vi "App_Remove User.vi"(8 "error in":errorcluster) -> (0 "error out":errorcluster)   [LabVIEW 2015, in "Application 1.lvlib"]
uses:
  Application 1.lvlib
  Data Def/App_Main Loop Queue Data.ctl
  Data Def/App_Subpanel Name.ctl
  Data Def/App_User Event Data.ctl
  Data Def/App_Config Method.ctl
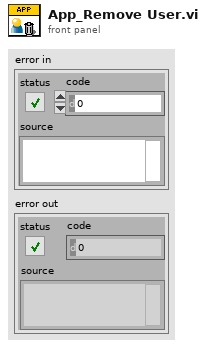
[diagram p1: front panel]
types:
  T1 = typedef "Application 1.lvlib/App_User Event Data.ctl" = cluster{"Command":string, "Data":variant}
  T2 = typedef "Application 1.lvlib/App_Subpanel Name.ctl" = enum16{"Main", "Menu", "User Registering", "User Setting", "Monitor", "Traning Mode", "Query Data", "Connect Setting"}
  T3 = typedef "Application 1.lvlib/App_Config Method.ctl" = enum16{"Get", "Put", "Load", "Save"}
  T4 = typedef "Application 1.lvlib/App_Main Loop Queue Data.ctl" = cluster{"Command":string, "Data":variant}
  T5 = typedef "Application 1.lvlib/App_Main Data.ctl" = cluster{"VI Refnum":refnum<vi>, "Subpanel":refnum<vi>, "Connection ID":refnum<k5>, "Meta data":T6[], "Main Queue":T8, "User Data":T9}
  T6 = typedef "stm_MetaElement.ctl" = cluster{"Name":T7}
  T7 = typedef "stm_MetaDataElement.ctl" = string
  T8 = typedef "Application 1.lvlib/App_Main Queue.ctl" = cluster{"Main Loop Queue":refnum<queue>}
  T9 = typedef "User Data.ctl" = cluster{"Name":string, "Email":string, "Phone Number":string, "User Picture":u32[][], "Last Login Time":timestamp}
  T10 = typedef "Application 1.lvlib/App_Configuration.ctl" = cluster{"Server IP":string, "User Name":string}
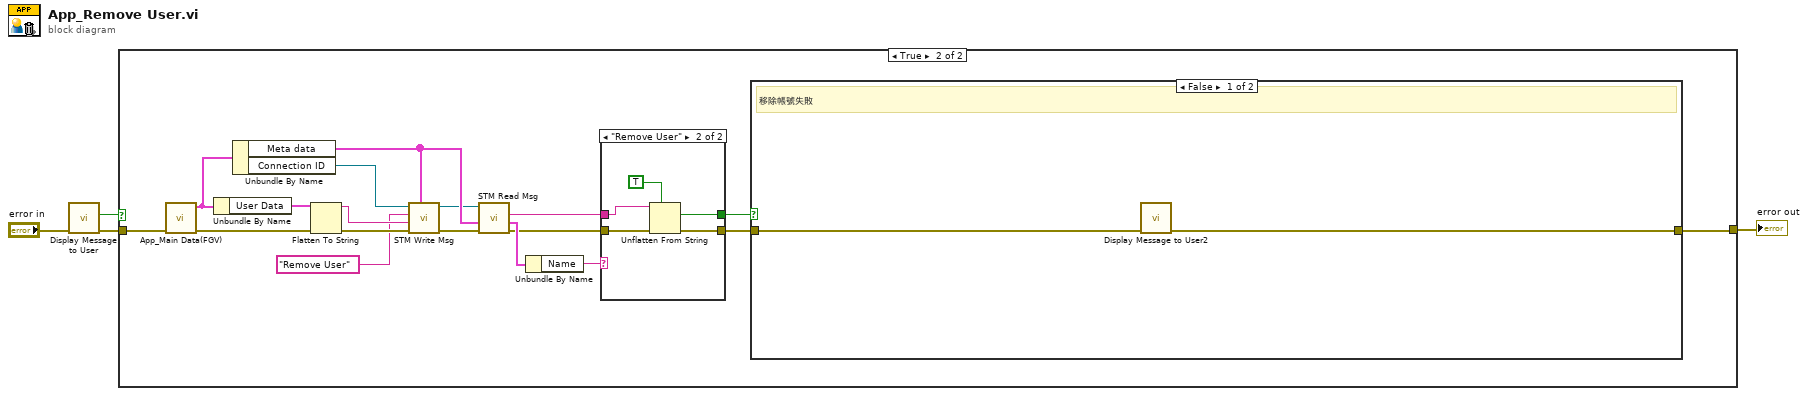
[diagram p0: block diagram]
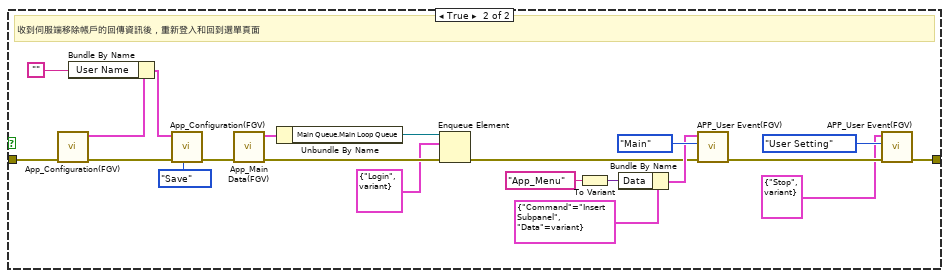
[diagram p3: hidden frame]
diagram:
  n1 = call "Display Message to User"("error in (no error)"="error in") -> ("error out"=w2:errorcluster, "OK"=w3:bool)  [unwired: 9 in]
  n2 = case shown="True" w3 {
    tunnel: w2 -> [w5 w23]
    tunnel: [w5 w6] -> w1
    frame False {
    }
    frame True {
      n3 = call "App_Main Data(FGV).vi"("error in"=w23) -> ("error out"=w22:errorcluster, "Main Data Out"=w20:T5)  [unwired: 9 in]
      n4 = Unbundle By Name(w20) -> ("User Data"=w21:T9)
      n5 = Unbundle By Name(w20) -> ("Meta data"=w14:T6[], "Connection ID"=w18:refnum<k5>)
      n6 = Flatten To String(anything=w21, error in (no error)=w22) -> (data string=w17:string, error out=w19:errorcluster)  [unwired: 2 in, 1 out]
      n7 = call "STM Write Msg.vi"("Meta data"=w14, "error in (no error)"=w19, "Data"=w17, "Name"="Remove User", "connection ID"=w18) -> ("error out"=w15:errorcluster, "connection ID out"=w13:refnum<k5>)  [unwired: 5 in]
      n8 = call "STM Read Msg.vi"("error in"=w15, "Meta data"=w14, "connection ID"=w13) -> ("error out"=w9:errorcluster, "Meta element"=w12:T6, "data string"=w10:string)  [unwired: 3 in, 3 out]
      n9 = Unbundle By Name(w12) -> ("Name"=w11:T7)
      n10 = case shown="\"Remove User\"" w11 {
        tunnel: w10 -> [_ w49]
        tunnel: w9 -> [_ w50]
        tunnel: [_ w47] -> w7
        tunnel: [_ w48] -> w8
        frame Default {
        }
        frame "Remove User" {
          n11 = Unflatten From String(type=TRUE, binary string=w49, error in (no error)=w50) -> (value=w48:bool, error out=w47:errorcluster)  [unwired: 2 in, 1 out]
        }
      }
      n12 = case shown="False" w8 {
        tunnel: w7 -> [w25 w28]
        tunnel: [w24 w26] -> w6
        frame False {
          # "移除帳號失敗"
          n13 = call "Display Message to User2"("error in (no error)"=w25) -> ("error out"=w24:errorcluster)  [unwired: 9 in, 1 out]
        }
        frame True {
          # "收到伺服端移除帳戶的回傳資訊後，重新登入和回到選單頁面"
          n14 = call "App_Configuration(FGV).vi"("error in"=w28) -> ("error out"=w35:errorcluster, "Configuration Out"=w36:T10)  [unwired: 9 in]
          n15 = Bundle By Name(cluster=w36, "User Name"="") -> (w34:T10)
          n16 = call "App_Configuration(FGV).vi"("Config Method(Get)"=App_Config_Method."Save", "error in"=w35, "Configuration In"=w34) -> ("error out"=w32:errorcluster)  [unwired: 7 in, 1 out]
          n17 = call "App_Main Data(FGV).vi"("error in"=w32) -> ("error out"=w45:errorcluster, "Main Data Out"=w46:T5)  [unwired: 9 in]
          n18 = Unbundle By Name(w46) -> ("Main Queue.Main Loop Queue"=w44:refnum<queue>)
          n19 = Enqueue Element(queue=w44, element=T4 {"Command"="Login", "Data"=variant}, error in (no error)=w45) -> (error out=w37:errorcluster)  [unwired: 1 in, 2 out]
          n20 = To Variant(anything="App_Menu") -> (Variant=w40:variant)
          n21 = Bundle By Name(cluster=T1 {"Command"="Insert Subpanel", "Data"=variant} ("User Event Data"), "Data"=w40) -> (w38:T1)
          n22 = call "APP_User Event(FGV).vi"("error in"=w37, "Subpanel Name"=App_Subpanel_Name."Main", "User Event Data"=w38) -> ("error out"=w31:errorcluster)  [unwired: 7 in, 1 out]
          n23 = call "APP_User Event(FGV).vi"("error in"=w31, "Subpanel Name"=App_Subpanel_Name."User Setting", "User Event Data"=T1 {"Command"="Stop", "Data"=variant}) -> ("error out"=w26:errorcluster)  [unwired: 7 in, 1 out]
        }
      }
    }
  }
  "error out" <- w1
